vi "Generate Token.vi"() -> (1 "Sync Token Refnum":T1)   [LabVIEW 2019, in "Sync Token.lvlib"]
doc: "Creates a new <b>Sync Token</b> instance. A Sync Token is a lightweight synchronisation primitive that can be used to coordinate execution between parallel LabVIEW code sections. This VI returns a unique token reference that can later be passed to <b>Wait on Token.vi</b> and <b>Set Token.vi</b>.\n\nUse this VI whenever you need to create a fresh token for a new synchronisation cycle or to replace a previously signalled token."
uses:
  Sync Token.lvlib
  Controls/Public/Sync Token Refnum.ctl
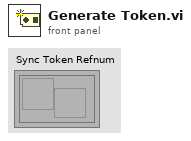
[diagram p1: front panel]
types:
  T1 = typedef "Sync Token.lvlib/Sync Token Refnum.ctl" = refnum<k1>
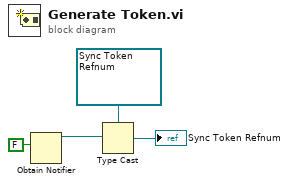
[diagram p0: block diagram]
diagram:
  n1 = Obtain Notifier(notification data type=FALSE) -> (notifier out=w3:refnum<notifier>)  [unwired: 3 in, 2 out]
  n2 = Type Cast(type=T1 refnum ("Sync Token Refnum"), x=w3) -> (*(type *) &x=→"Sync Token Refnum":T1)
